vi "Belt Speed FG.vi"(1 "Speed In":dbl format="%#_13g", 2 "Menu":T1) -> (0 "Speed Out":dbl)   [LabVIEW 2013]
uses:
  typedefs/fg_typedef.ctl
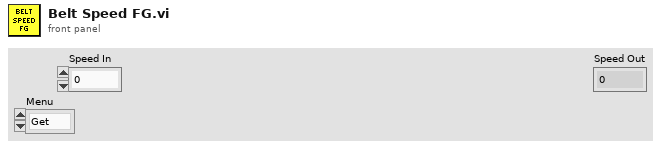
[diagram p1: front panel]
types:
  T1 = typedef "fg_typedef.ctl" = enum16{"Get", "Set"}
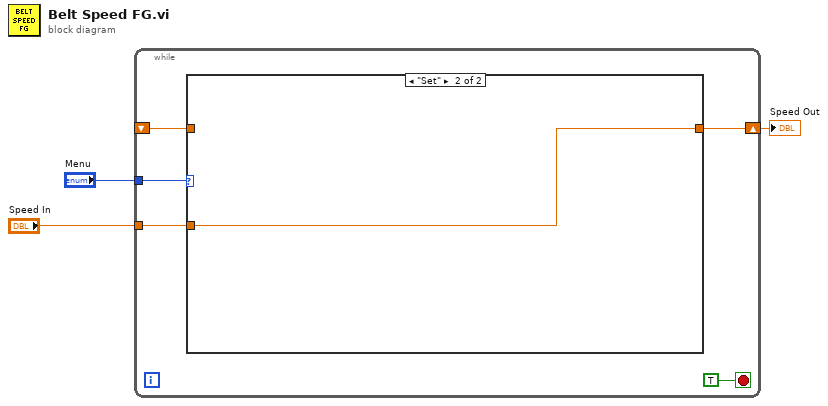
[diagram p0: block diagram]
diagram:
  n1 = while {
    tunnel: "Menu" -> [w7]
    shift-right: [w6] -> w1
    shift-left: _ -> [w5]
    tunnel: "Speed In" -> [w4]
    stop <- TRUE stop-if-true
    n2 = case shown="\"Set\"" w7 {
      tunnel: [w9 w10] -> w6
      tunnel: w5 -> [w9 _]
      tunnel: w4 -> [_ w10]
      frame "Get", Default {
      }
      frame "Set" {
      }
    }
  }
  "Speed Out" <- w1
